vi "calculate voltages from artificial forces.vi"(2 "offsets":dbl[](array[numeric]), 3 "Mean Trap Positions (nm)":T2={"T1 X"=3248.000000000121, "T2 X"=6090.0, "T3 X"=4120.979470198669, "T3 Y"=2049.2494705038607} {"T3 Y" format="%#_6f"; "T3 X" format="%#_6f"; "T2 X" format="%#_6f"; "T1 X" format="%#_6f"}, 4 "T3 calibration":T3={"alpha_x (nm/V)"=710.5060104266419, "offset_x (mV)"=-36.090285107024734, "kappa_x (pN/nm)"=0.3159761713941174, "alpha_y (nm/V)"=753.1143150189287, "kappa_y (pN/nm)"=0.2993483344894904, "offset_y (mV)"=-18.775215803744803} {"offset_y (mV)" format="%#_2g"; "kappa_y (pN/nm)" min=0.0 step=0.001 format="%#_2g"; "alpha_y (nm/V)" step=10.0 format="%#_3g"; "kappa_x (pN/nm)" min=0.0 step=0.001 format="%#_2g"; "offset_x (mV)" format="%#_2g"; "alpha_x (nm/V)" step=10.0 format="%#_3g"}, 5 "T2 calibration":T3={"alpha_x (nm/V)"=561.9370989425553, "offset_x (mV)"=49.70435379070299, "kappa_x (pN/nm)"=0.4022490871584769, "alpha_y (nm/V)"=671.0236177196408, "kappa_y (pN/nm)"=0.4165200151330455, "offset_y (mV)"=-133.18321148420554} {"offset_y (mV)" format="%#_2g"; "kappa_y (pN/nm)" min=0.0 step=0.001 format="%#_2g"; "alpha_y (nm/V)" step=10.0 format="%#_3g"; "kappa_x (pN/nm)" min=0.0 step=0.001 format="%#_2g"; "offset_x (mV)" format="%#_2g"; "alpha_x (nm/V)" step=10.0 format="%#_3g"}, 6 "T1 calibration":T3={"alpha_x (nm/V)"=556.2687255652412, "offset_x (mV)"=54.165144990257225, "kappa_x (pN/nm)"=0.4102591892061342, "alpha_y (nm/V)"=683.0922954326962, "kappa_y (pN/nm)"=0.4103334611769005, "offset_y (mV)"=-94.27748475526903} {"offset_y (mV)" format="%#_2g"; "kappa_y (pN/nm)" min=0.0 step=0.001 format="%#_2g"; "alpha_y (nm/V)" step=10.0 format="%#_3g"; "kappa_x (pN/nm)" min=0.0 step=0.001 format="%#_2g"; "offset_x (mV)" format="%#_2g"; "alpha_x (nm/V)" step=10.0 format="%#_3g"}, 7 "Desired forces (pN)":T4={"F1x"=0.0605018, "F1y"=0.0, "F2x"=0.0507675, "F2y"=0.0}) -> (0 "ratio":dbl, 1 "Output displacements":T1={"A_X"=0.0605018, "A_Y"=0.0, "B_X"=0.0507675, "B_Y"=0.0, "C_X"=0.0, "C_Y"=0.0})   [LabVIEW 2014]
uses:
  <vilib>/imath/engines/lvmath2/RunTimeEngine/NodeEndStatement/NIMS_NodeEndStatement_Output.vi
  <instcachedir>/0/NIMS_NodeEndStatement_Output_53EC0D466D134D7ABD903AC30B43404B.lvgen/NIMS_NodeEndStatement_Output_53EC0D466D134D7ABD903AC30B43404B_001.vi
  <vilib>/imath/engines/lvmath2/RunTimeEngine/ErrorHandling/NIMS_Finalize Error.vi
panel:
  out "Force (pN)":T1={"A_X"=0.0605018, "A_Y"=0.0, "B_X"=0.0507675, "B_Y"=0.0, "C_X"=0.0, "C_Y"=0.0}
  in  "Displacments":T1={"A_X"=0.0605018, "A_Y"=0.0, "B_X"=0.0507675, "B_Y"=0.0, "C_X"=0.0, "C_Y"=0.0}
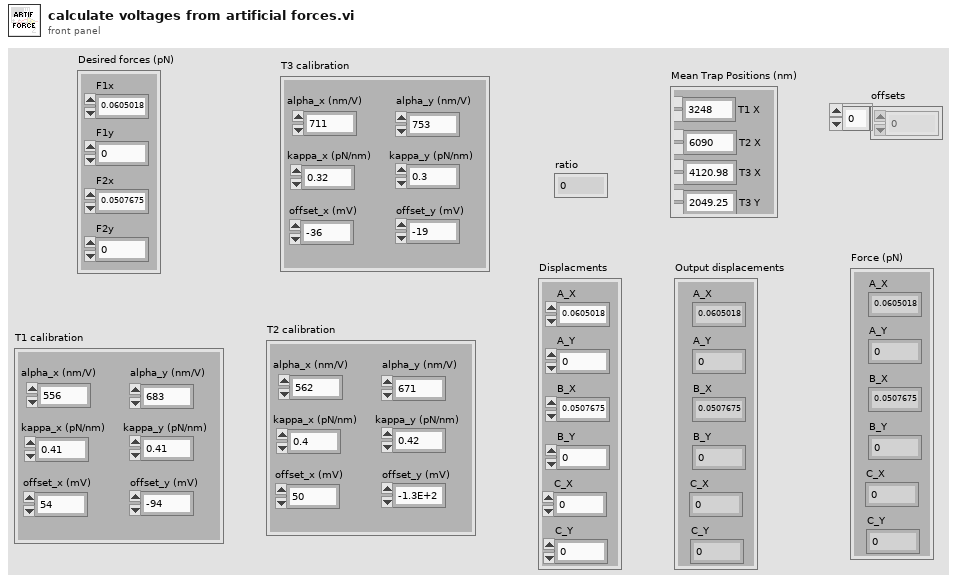
[diagram p1: front panel]
types:
  T1 = cluster{"A_X":dbl, "A_Y":dbl, "B_X":dbl, "B_Y":dbl, "C_X":dbl, "C_Y":dbl}
  T2 = cluster{"T1 X":dbl, "T2 X":dbl, "T3 X":dbl, "T3 Y":dbl}
  T3 = cluster{"alpha_x (nm/V)":dbl, "offset_x (mV)":dbl, "kappa_x (pN/nm)":dbl, "alpha_y (nm/V)":dbl, "kappa_y (pN/nm)":dbl, "offset_y (mV)":dbl}
  T4 = cluster{"F1x":dbl, "F1y":dbl, "F2x":dbl, "F2y":dbl}
  T5 = cluster{"offsets[0]":dbl, "offsets[1]":dbl, "offsets[2]":dbl, "offsets[3]":dbl, "offsets[4]":dbl, "offsets[5]":dbl}
  T6 = cluster{"F1x":dbl, "F1y":dbl, "F2x":dbl, "F2y":dbl, "F3x":dbl, "F3y":dbl}
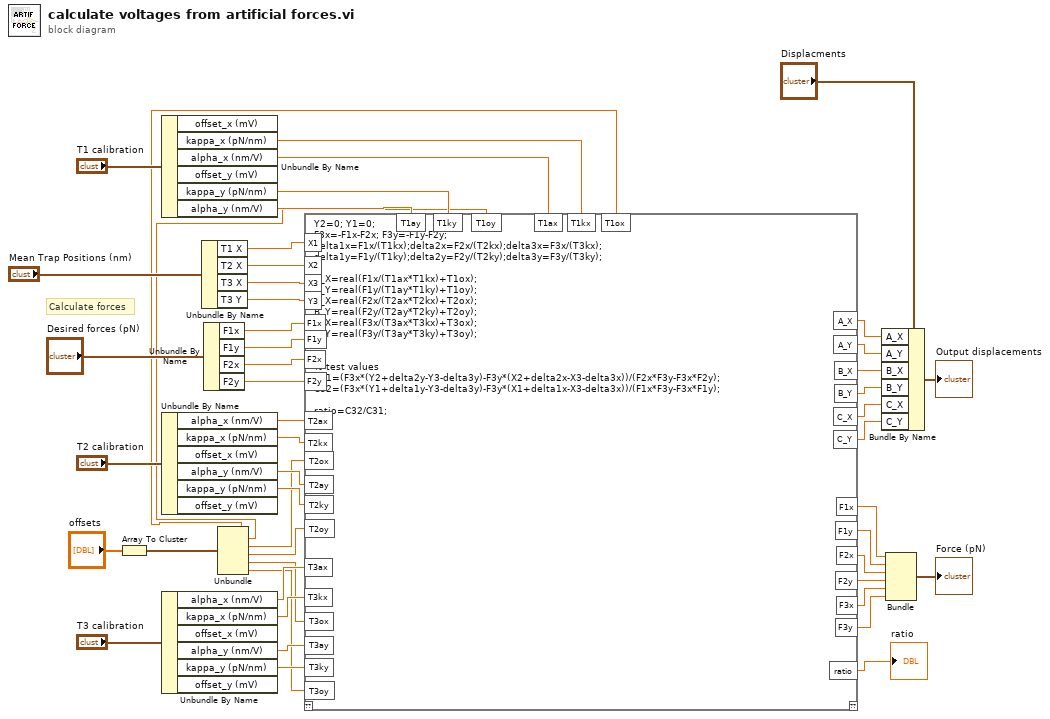
[diagram p0: block diagram]
diagram:
  # "Calculate forces"
  n1 = Array To Cluster(array="offsets") -> (cluster=w10:T5)
  n2 = Unbundle By Name("T1 calibration") -> ("kappa_x (pN/nm)"=w38:dbl, "alpha_x (nm/V)"=w37:dbl, "kappa_y (pN/nm)"=w36:dbl, "alpha_y (nm/V)"=w35:dbl)  [unwired: 2 out]
  n3 = Unbundle By Name("T2 calibration") -> ("alpha_x (nm/V)"=w34:dbl, "kappa_x (pN/nm)"=w33:dbl, "alpha_y (nm/V)"=w32:dbl, "kappa_y (pN/nm)"=w31:dbl)  [unwired: 2 out]
  n4 = Unbundle By Name("T3 calibration") -> ("alpha_x (nm/V)"=w30:dbl, "kappa_x (pN/nm)"=w29:dbl, "alpha_y (nm/V)"=w28:dbl, "kappa_y (pN/nm)"=w27:dbl)  [unwired: 2 out]
  n5 = Unbundle By Name("Mean Trap Positions (nm)") -> ("T1 X"=w45:dbl, "T2 X"=w44:dbl, "T3 X"=w3:dbl, "T3 Y"=w2:dbl)
  n6 = Unbundle By Name("Desired forces (pN)") -> ("F1x"=w43:dbl, "F1y"=w42:dbl, "F2x"=w41:dbl, "F2y"=w40:dbl)
  n7 = Unbundle(w10) -> ("offsets[0]"=w9:dbl, "offsets[1]"=w8:dbl, "offsets[2]"=w7:dbl, "offsets[3]"=w6:dbl, "offsets[4]"=w5:dbl, "offsets[5]"=w4:dbl)
  n8 = mathscript code="Y2=0; Y1=0;\nF3x=-F1x-F2x; F3y=-F1y-F2y;\ndelta1x=F1x/(T1kx);delta2x=F2x/(T2kx);delta3x=F3x/(T3kx);\ndelta1y=F1y/(T1ky);delta2y=F2y/(T2ky);delta3y=F3y/(T3ky);\n\nA_X=real(F1x/(T1ax*T1kx)+T1ox);\nA_Y=real(F1y/(T1ay*T1ky)+T1oy);\nB_X=real(F2x/(T2ax*T2kx)+T2ox);\nB_Y=real(F2y/(T2ay*T2ky)+T2oy);\nC_X=real(F3x/(T3ax*T3kx)+T3ox);\nC_Y=real(F3y/(T3ay*T3ky)+T3oy);\n\n\n% test values\nC31=(F3x*(Y2+delta2y-Y3-delta3y)-F3y*(X2+delta2x-X3-delta3x))/(F2x*F3y-F3x*F2y);\nC32=(F3x*(Y1+delta1y-Y3-delta3y)-F3y*(X1+delta1x-X3-delta3x))/(F1x*F3y-F3x*F1y);\n\nratio=C32/C31;"("X1"=w45, "X2"=w44, "F1x"=w43, "F1y"=w42, "F2x"=w41, "F2y"=w40, "T1ax"=w37, "T1kx"=w38, "T1ox"=w9, "T1ay"=w35, "T1ky"=w36, "T1oy"=w8, "T2ax"=w34, "T2kx"=w33, "T2ox"=w7, "T2ay"=w32, "T2ky"=w31, "T2oy"=w6, "T3ax"=w30, "T3kx"=w29, "T3ox"=w5, "T3ay"=w28, "T3ky"=w27, "T3oy"=w4, "X3"=w3, "Y3"=w2) -> ("A_X"=w25:dbl, "A_Y"=w24:dbl, "B_X"=w23:dbl, "B_Y"=w22:dbl, "C_X"=w21:dbl, "C_Y"=w20:dbl, "F1x"=w18:dbl, "F2x"=w12:dbl, "F1y"=w13:dbl, "F2y"=w17:dbl, "F3x"=w16:dbl, "F3y"=w15:dbl, "ratio"=→"ratio":dbl)  [unwired: 1 in, 1 out]
  n9 = Bundle By Name(cluster="Displacments", "A_X"=w25, "A_Y"=w24, "B_X"=w23, "B_Y"=w22, "C_X"=w21, "C_Y"=w20) -> (→"Output displacements":T1)
  n10 = Bundle("F1x"=w18, "F1y"=w13, "F2x"=w12, "F2y"=w17, "F3x"=w16, "F3y"=w15) -> (→"Force (pN)":T6)  [unwired: 1 in]
